vi "gds_rx_rcv.vi"(8 "error in (no error)":errorcluster, 10 "HW parameters In":T2={"Device IP Address"="192.168.11.6", "Active Antenna"="RX1", "Carrier Frequency (Hz)"=915000000.0, "Gain (dB)"=10.0, "Trigger Level"=0.01, "Bandwidth (Hz)"=40000000.0, "Reference Position (%)"=10.0, "Capture Time (s)"=0.0004, "Simulate"=FALSE} {"Capture Time (s)" format="%.2p"; "Bandwidth (Hz)" format="%.2p"; "Trigger Level" format="%#.3p"; "Gain (dB)" format="%.2f"; "Carrier Frequency (Hz)" format="%.2p"}, 11 "Modulation Parameters":T1) -> (0 "error out":errorcluster, 1 "Received IQ waveform":cluster{"t0":dbl, "dt":dbl, "Y":cdb[]} {"Y" format="%.2g"; "dt" format="%.2g"; "t0" format="%.2g"}, 2 "HW parameters Out":T2={"Device IP Address"="192.168.11.6", "Active Antenna"="RX1", "Carrier Frequency (Hz)"=915000000.0, "Gain (dB)"=10.0, "Trigger Level"=0.01, "Bandwidth (Hz)"=40000000.0, "Reference Position (%)"=10.0, "Capture Time (s)"=0.0004, "Simulate"=FALSE} {"Capture Time (s)" format="%.2p"; "Bandwidth (Hz)" format="%.2p"; "Trigger Level" format="%#.3p"; "Gain (dB)" format="%.2f"; "Carrier Frequency (Hz)" format="%.2p"}, 3 "Modulation Parameters Out":T1, 5 "Packet Detected":bool)   [LabVIEW 2012]
uses:
  EE 497/LABS/SDR/control_type_defs.llb/rx_hw params.ctl
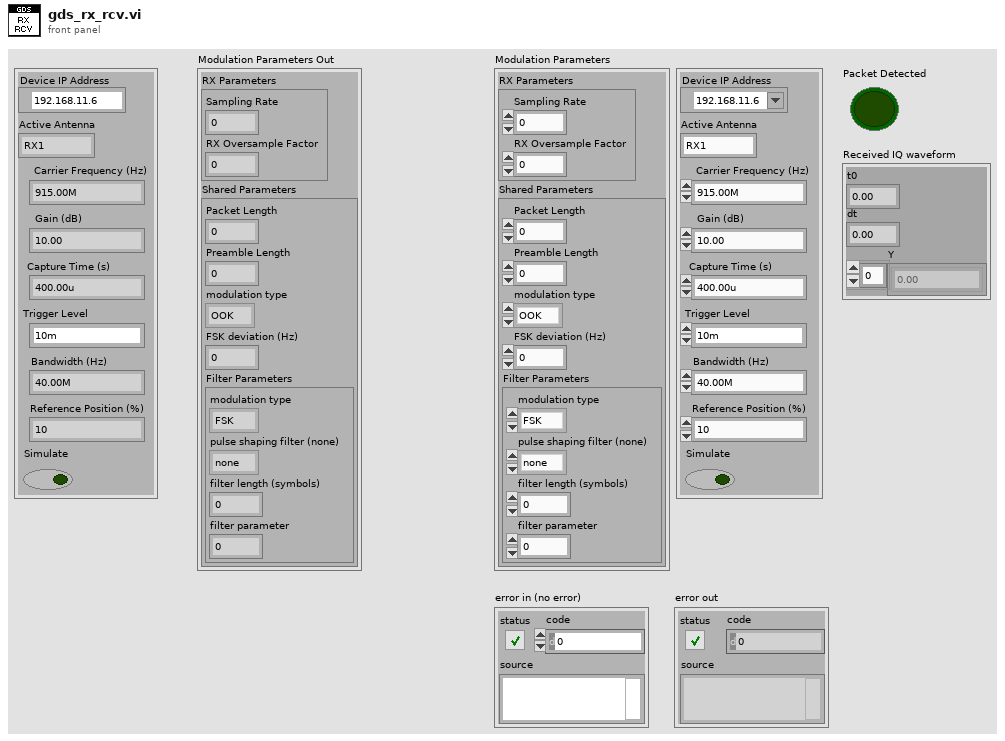
[diagram p1: front panel]
types:
  T1 = cluster{"RX Parameters":cluster{"Sampling Rate":dbl, "RX Oversample Factor":i32}, "Shared Parameters":cluster{"Packet Length":i32, "Preamble Length":i32, "modulation type":enum16{"OOK", "FSK", "PSK", "QAM", "MSK", "PAM", "ASK", "CPM"}, "FSK deviation (Hz)":dbl, "Filter Parameters":cluster{"modulation type":enum16{"FSK", "PSK", "QAM", "MSK", "PAM", "ASK", "CPM"}, "pulse shaping filter (none)":enum16{"none", "Raised Cosine", "Root Raised Cos", "Gaussian"}, "filter length (symbols)":i32, "filter parameter":dbl}}}
  T2 = typedef "rx_hw params.ctl" = cluster{"Device IP Address":refnum<k15>, "Active Antenna":string, "Carrier Frequency (Hz)":dbl, "Gain (dB)":dbl, "Trigger Level":dbl, "Bandwidth (Hz)":dbl, "Reference Position (%)":dbl, "Capture Time (s)":dbl, "Simulate":bool}
  T3 = cluster{"Sampling Rate":dbl, "RX Oversample Factor":i32}
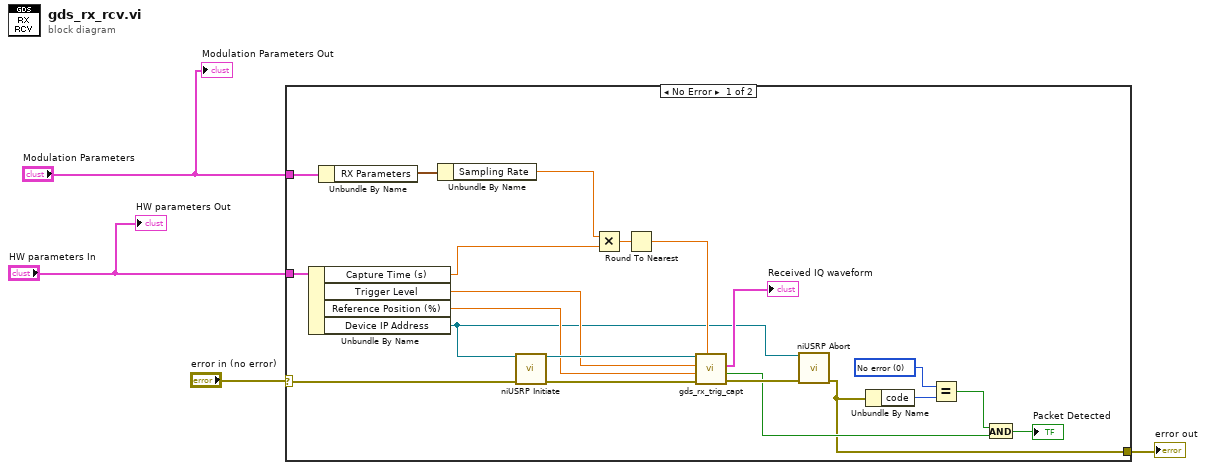
[diagram p0: block diagram]
diagram:
  n1 = case shown="No Error" "error in (no error)" {
    selector: "error in (no error)" -> [w22 w26]
    tunnel: [w5 w26] -> w3
    tunnel: "Modulation Parameters" -> [w25 _]
    tunnel: "HW parameters In" -> [w23 _]
    frame No Error {
      w9 = 0 items=["No error", "Argument error", "Memory is full", "Out of zone", "End of file", "File already open", "Generic file I/O error", "File not found", "File permission error", "Disk is full", "Duplicate path", "Too many files open", "System feature not enabled", "Resource file not found", "Cannot add resource", "Resource not found", "Image not found", "Image memory error", "Pen does not exist", "Config type invalid", "Config token not found", "Config parse error", "Config memory error", "Bad external code format", "Bad external code offset", "External code not present", "Null window", "Destroy window error", "Null menu", "Print aborted", "Bad print record", "Print driver error", "Windows error during printing", "Memory error during printing", "Print dialog error", "Generic print error", "Invalid device refnum", "Device not found", "Device parameter error", "Device unit error", "Cannot open device", "Device call aborted", "Generic error", "Cancelled by user", "Object ID too low", "Object ID too high", "Object not in heap", "Unknown heap", "Unknown object (invalid DefProc)", "Unknown object (DefProc not in table)", "Message out of range", "Invalid (null) method", "Unknown message", "Manager call not supported", "Bad address", "Network operation in progress", "Network operation timed out", "Connection is busy", "Network attribute not supported", "Network error", "Address in use", "System out of memory", "Connection aborted", "Connection refused", "Not connected", "Already connected", "Connection closed", "Initialization error (interapplication manager)", "Bad occurrence", "Wait on unbound occurrence handler", "Occurrence queue overflow", "Datalog type conflict", "Unused", "Unrecognized type (interapplication manager)", "Memory corrupt", "Failed to make temporary DLL", "Old CIN version", "Drag socket not found", "Failed to load drop-object", "Failed to register OLE object", "Failed to release OLE object", "Format specifier type mismatch", "Unknown format specifier", "Too few format specifiers", "Too many format specifiers", "Scan failed", "Newer CIN version", "Error converting to variant", "Runtime menu error", "Password tampered", "Variant attribute not found", "Incompatible variant data type", "Event data is not available", "Event Store is not present", "Occurrence is not found", "Event Queue is not created", "Event info is not available in the type library", "Refnum passed is NULL", "Error retrieving Class GUID", "Error retrieving CoClass GUID", "Error retrieving TypeLib GUID.", "Bad built application magic bytes.", "Specific driver is different from the specific driver associated with the Logical Name.", "There is no session opened to the class driver.", "Max Error", "MAX - Error with config objects", "MAX - Error loading configuration", "MAX - Group not supported", "Singlecast connections can not send to multicast addresses.", "Multicast connections can not send to singlecast addresses.", "Specified IP address not in multicast address range.", "Attempt to write to read-only multicast connection.", "Attempt to read from write-only multicast connection.", "The buffer used to receive a datagram was smaller than the datagram itself"]
      n2 = Unbundle By Name(w23) -> ("Capture Time (s)"=w21:dbl, "Trigger Level"=w16:dbl, "Reference Position (%)"=w15:dbl, "Device IP Address"=w12:refnum<k15>)
      n3 = Unbundle By Name(w25) -> ("RX Parameters"=w24:T3)
      n4 = Unbundle By Name(w24) -> ("Sampling Rate"=w20:dbl)
      n5 = call <instrlib>:"niUSRP Initiate.vi"("session handle"=w12, "error in (no error)"=w22) -> ("session handle out"=w17:refnum<k15>, "error out"=w18:errorcluster)  [unwired: 12 in]
      n6 = Multiply(x=w20, y=w21) -> (x*y=w19:dbl)
      n7 = Round To Nearest(number=w19) -> (nearest integer value=w14:dbl)
      n8 = call "gds_rx_trig_capt.vi"("number of samples"=w14, "error in (no error)"=w18, "reference\nposition"=w15, "trigger level"=w16, "session handle"=w17) -> ("error out"=w11:errorcluster, "packet found"=w7:bool, "IQ Waveform"=→"Received IQ waveform":cluster{"t0":dbl, "dt":dbl, "Y":cdb[]})  [unwired: 3 in, 1 out]
      n9 = call <instrlib>:"niUSRP Abort.vi"("session handle"=w12, "error in (no error)"=w11) -> ("error out"=w5:errorcluster)  [unwired: 12 in, 1 out]
      n10 = Unbundle By Name(w5) -> ("code"=w10:i32)
      n11 = Equal?(x=w9, y=w10) -> (x = y?=w8:bool)
      n12 = And(x=w8, y=w7) -> (x .and. y?=→"Packet Detected":bool)
    }
    frame Error {
    }
  }
  "error out" <- w3
  "HW parameters Out" <- "HW parameters In"
  "Modulation Parameters Out" <- "Modulation Parameters"
